vi "PDF Table Facade.vi"(0 "Data In":T5, 2 "Display State In":T3, 3 "Container State":T4) -> (6 "Data Out":T5, 7 "Display State Out":T3, 8 "Action":T2)   [LabVIEW 2012, in "PDF Table XControl.xctl"]
uses:
  PDF Table XControl.xctl
  PDF Table Data.ctl
  C:/Users/MaxCorp/Documents/TopPerm - Base/DLL/itextsharp.dll
  DLL/itextsharp.dll
  <vilib>/_xctls/Container State.ctl
  PDF Table State.ctl
  <vilib>/_xctls/Action.ctl
  Table ring.ctl
  <vilib>/Utility/miscctls.llb/LVPointTypeDef.ctl
  <vilib>/_xctls/XControlSupport.lvlib
panel:
  in  "Ring":T1
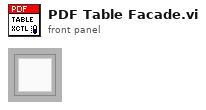
[diagram p1: front panel]
types:
  T1 = typedef "Table ring.ctl" = u16
  T2 = typedef "XControlSupport.lvlib/Action.ctl" = cluster{"Data Changed?":bool, "State Changed?":bool, "Action Name":string}
  T3 = typedef "PDF Table XControl.xctl/PDF Table State.ctl" = cluster{"Action":string, "Clear":bool}
  T4 = typedef "XControlSupport.lvlib/Container State.ctl" = cluster{"Indicator?":bool, "Run Mode?":bool, " Refnum":refnum<vi>}
  T5 = typedef "PDF Table XControl.xctl/PDF Table Data.ctl" = cluster{"PDFTable ref":refnum<k24>, "columnWidth (points)":sgl[], "Title 1D":string[], "Table Datas 2D":string[][], "Image to Add with refnum[ ]":cluster{"Image name":string, "InstanceImage":refnum<k24>}[]}
  T6 = typedef "LVPointTypeDef.ctl" = cluster{"Horizontal":i16, "Vertical":i16}
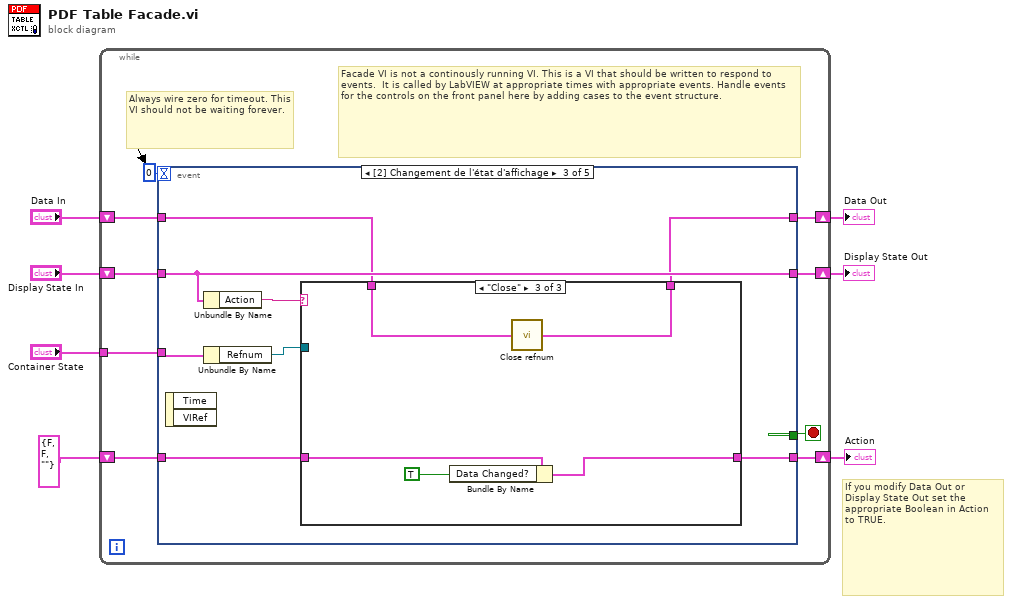
[diagram p0: block diagram]
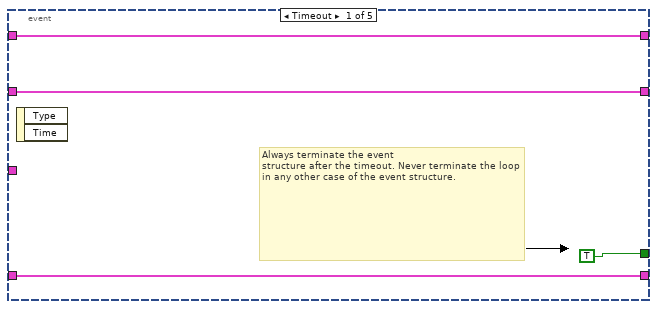
[diagram p2: hidden frame]
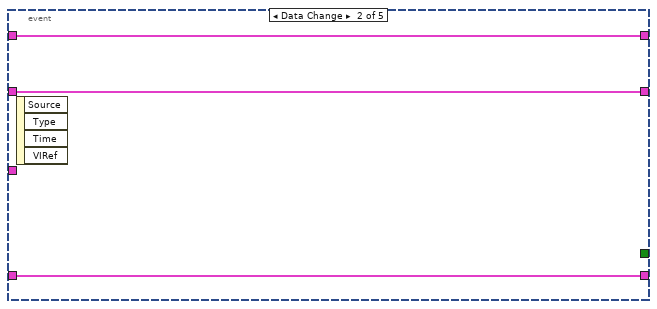
[diagram p3: hidden frame]
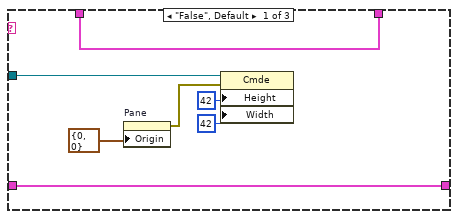
[diagram p4: hidden frame]
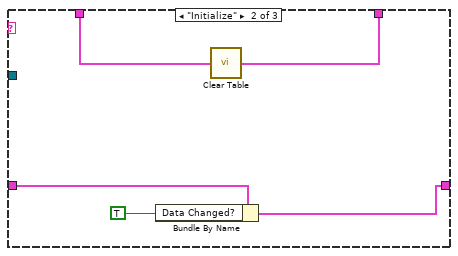
[diagram p5: hidden frame]
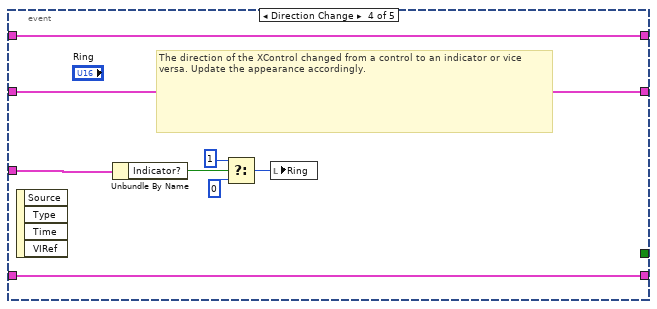
[diagram p6: hidden frame]
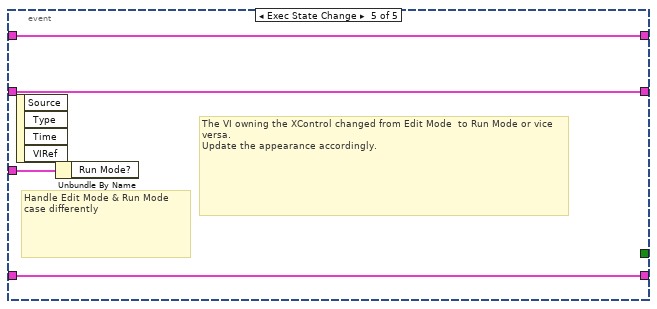
[diagram p7: hidden frame]
diagram:
  # "If you modify Data Out or\nDisplay State Out set the\nappropriate Boolean in Action\nto TRUE."
  n1 = while {
    shift-right: [w15] -> w4
    shift-left: "Display State In" -> [w16]
    tunnel: "Container State" -> [w12]
    shift-right: [w8] -> w7
    shift-left: "Data In" -> [w11]
    shift-right: [w9] -> w2
    shift-left: T2 {"Data Changed?"=FALSE, "State Changed?"=FALSE, "Action Name"=""} ("Action") -> [w10]
    stop <- w14 stop-if-true
    # "Facade VI is not a continously running VI. This is a VI that should be written to respond to events.  It is called by LabVIEW at appropriate times with appropriate events. Handle events for the controls on the front panel here by adding cases to the event structure."
    # "Always wire zero for timeout. This\nVI should not be waiting forever."
    n2 = event shown="[2] Changement de l'état d'affichage" {
      selector: _ -> [_ _ _ _ _]
      dyn-events: _ -> [_ _ _ _ _]
      timeout: 0 -> [_ _ _ _ _]
      tunnel: w16 -> [w18 w23 w30 w55 w59]
      tunnel: [w18 w23 w30 w55 w59] -> w15
      tunnel: [TRUE _ _ _ _] -> w14
      tunnel: w12 -> [_ _ w31 w56 w60]
      tunnel: w11 -> [w17 w22 w26 w54 w58]
      tunnel: [w19 w21 w28 w53 w57] -> w9
      tunnel: w10 -> [w19 w21 w27 w53 w57]
      tunnel: [w17 w22 w25 w54 w58] -> w8
      event Timeout {
        # "Always terminate the event\nstructure after the timeout. Never terminate the loop in any other case of the event structure."
        n3 = event-data() -> ()  [unwired: 3 out]
      }
      event Data Change {
        n4 = event-data() -> ()  [unwired: 5 out]
      }
      event Display State Change {
        n5 = event-data() -> ()  [unwired: 3 out]
        n6 = Unbundle By Name(w30) -> ("Action"=w29:string)
        n7 = Unbundle By Name(w31) -> ("Refnum"=w24:refnum<vi>)
        n8 = case shown="\"Close\"" w29 {
          tunnel: [w37 w41 w47] -> w28
          tunnel: w27 -> [w37 w42 w48]
          tunnel: w26 -> [w36 w40 w44]
          tunnel: [w36 w39 w45] -> w25
          tunnel: w24 -> [w35 _ _]
          frame "False", Default {
            n9 = property on="Pane" class="Pann"("Origin"=T6 {"Horizontal"=0, "Vertical"=0}) -> (error out=w34:errorcluster)  [unwired: 2 in, 1 out]
            n10 = property class="Cmde"(reference=w35, error in=w34, "Height"=u32 42 ("XControl:Container Bounds:Height"), "Width"=u32 42 ("XControl:Container Bounds:Width")) -> ()  [unwired: 2 out]
          }
          frame "Initialize" {
            n11 = Bundle By Name(cluster=w42, "Data Changed?"=TRUE) -> (w41:T2)
            n12 = call "Clear Table.vi"("Data IN"=w40) -> ("Data OUT"=w39:T5)
          }
          frame "Close" {
            n13 = Bundle By Name(cluster=w48, "Data Changed?"=TRUE) -> (w47:T2)
            n14 = call "Close refnum.vi"("Data IN"=w44) -> ("Data OUT"=w45:T5)
          }
        }
      }
      event Direction Change {
        # "The direction of the XControl changed from a control to an indicator or vice versa. Update the appearance accordingly."
        n15 = event-data() -> ()  [unwired: 5 out]
        n16 = Unbundle By Name(w56) -> ("Indicator?"=w52:bool)
        n17 = Select(t=T1 1 ("Ring"), s=w52, f=T1 0 ("Ring")) -> (s? t:f=w51:T1)
        n18 = local write "Ring"(w51) -> ()
      }
      event Exec State Change {
        # "The VI owning the XControl changed from Edit Mode  to Run Mode or vice versa.\nUpdate the appearance accordingly."
        # "Handle Edit Mode & Run Mode\ncase differently"
        n19 = event-data() -> ()  [unwired: 5 out]
        n20 = Unbundle By Name(w60) -> ()  [unwired: 1 out]
      }
    }
  }
  "Display State Out" <- w4
  "Data Out" <- w7
  "Action" <- w2
